vi "Main RT.vi"() -> ()   [LabVIEW 2021]
uses:
  <vilib>/FPGAPlugInAG/myRIO-1900/niLvFpga_Open_myRIO-1900.vi
  <vilib>/rvi/interface/common/dynamic/niFpgaDynamicAddResources.vi
  <vilib>/FPGAPlugInAG/Dynamic/niLvFpga_Run_Dynamic.vi
  <vilib>/Utility/error.llb/Error Cluster From Error Code.vi
  <vilib>/rvi/errors/niLvFpgaAdjustHostInterfaceError.vi
  <vilib>/FPGAPlugInAG/Dynamic/niLvFpga_Close_Dynamic.vi
  <vilib>/rvi/interface/nirviOpenFPGA/nirviOpenFPGA.xnode
  FPGA Bitfiles/tdmsproject_FPGATarget_MainFPGA_3ScZJD+QSjs.lvbitx
  <vilib>/rvi/interface/nirviMethod/nirviMethod.xnode
  <vilib>/rvi/interface/nirviReadWriteControl/nirviReadWriteControl.xnode
  <vilib>/rvi/interface/nirviCloseFPGA/nirviCloseFPGA.xnode
  NiFpgaLv.dll
  <vilib>/rvi/interface/Simulation/niFpgaSimulationCallBeginRW.vi
panel:
  in  "LED0":bool
  in  "stop":bool
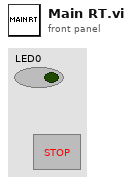
[diagram p1: front panel]
types:
  T1 = enum16{"open", "open or create", "create or replace", "create", "open (read-only)"}
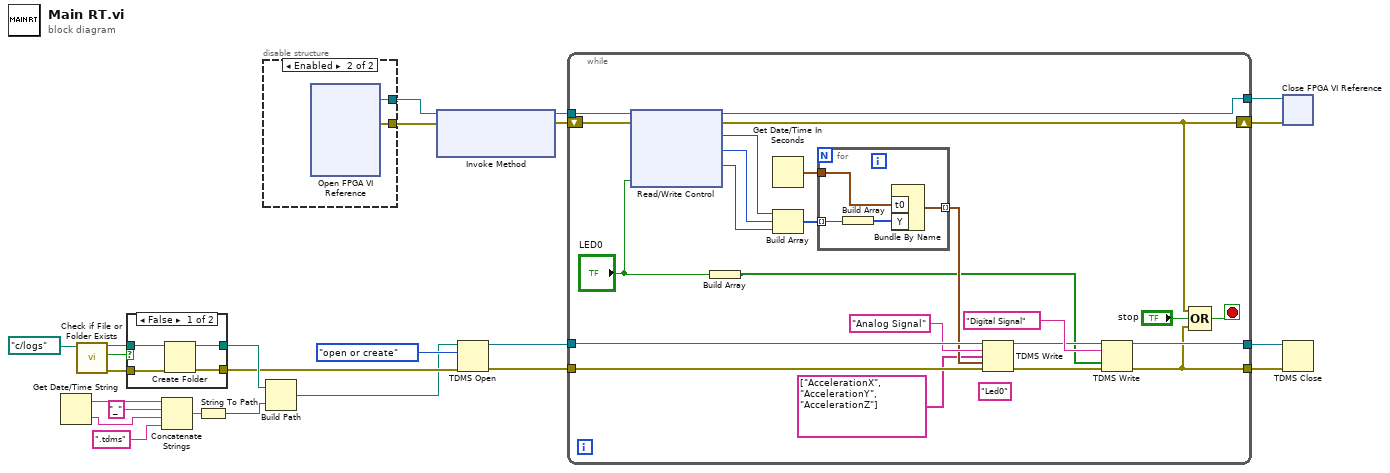
[diagram p0: block diagram]
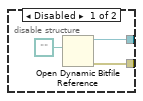
[diagram p3: hidden frame]
diagram:
  n1 = Get Date/Time String() -> (date string=w6:string, time string=w4:string)  [unwired: 3 in]
  n2 = call <vilib>:"Check if File or Folder Exists.vi"("path"=path "c:/logs" ("file path")) -> ("error out"=w10:errorcluster, "file or folder exists?"=w11:bool, "dup path"=w12:path)  [unwired: 8 in]
  n3 = case shown="False" w11 {
    tunnel: w12 -> [w28 w30]
    tunnel: [w27 w30] -> w9
    tunnel: [w26 w29] -> w8
    tunnel: w10 -> [w25 w29]
    frame False {
      n4 = Create Folder(path (use dialog)=w28, error in=w25) -> (created path=w27:path, error out=w26:errorcluster)  [unwired: 1 in, 1 out]
    }
    frame True {
    }
  }
  n5 = Concatenate Strings(w6, "_" ("string"), w4, ".tdms" ("string")) -> (w3:string)
  n6 = String To Path(string=w3) -> (path=w1:path)
  n7 = disable-structure shown="Enabled" {
    disable-tunnel: [w33 w34] -> w23
    disable-tunnel: [w32 w35] -> w22
    frame Disabled {
      n8 = Open Dynamic Bitfile Reference(1:path "" ("Bitfile path")) -> (5:w33:refnum<k20>, 8:w32:errorcluster)  [unwired: 4 in]
    }
    frame Enabled {
      n9 = xnode "Open FPGA VI Reference"() -> ("FPGA VI Reference Out"=w34:refnum<k20>, "error out"=w35:errorcluster)  [unwired: 2 in]
    }
  }
  n10 = Build Path(base path=w9, name or relative path=w1) -> (appended path=w7:path)
  n11 = xnode "Invoke Method"("FPGA VI Reference In"=w23, "error in"=w22) -> ("FPGA VI Reference Out"=w24:refnum<k20>, "error out"=w21:errorcluster)  [unwired: 1 in]
  n12 = TDMS Open(8:w8, 10:T1."open or create" ("operation (0:open)"), 11:w7) -> (0:w17:errorcluster, 3:w18:refnum<k34>)  [unwired: 4 in]
  n13 = while {
    tunnel: w24 -> [w58]
    shift-right: [w38] -> w20
    shift-left: w21 -> [w57]
    tunnel: [w56] -> w19
    tunnel: w18 -> [w55]
    tunnel: w17 -> [w54]
    tunnel: [w50] -> w16
    tunnel: [w36] -> w15
    stop <- w39 stop-if-true
    (unwired) "Led0" ("channel name(s) in (Untitled)")
    n14 = xnode "Read/Write Control"("FPGA VI Reference In"=w58, "error in"=w57, "LED0"="LED0") -> ("FPGA VI Reference Out"=w56:refnum<k20>, "error out"=w38:errorcluster, "AccelerationX"=w48:i16, "AccelerationY"=w47:i16, "AccelerationZ"=w43:i16)
    n15 = Build Array("LED0") -> (w41:bool[])
    n16 = Get Date/Time In Seconds() -> (seconds since 1Jan1904=w44:timestamp)
    n17 = Build Array(w48, w47, w43) -> (w46:i16[])
    n18 = for {
      tunnel: w46 -> [w60] mode=indexing
      tunnel: [w62] -> w45 mode=indexing
      tunnel: w44 -> [w61]
      n19 = Build Array(w60) -> (w59:i16[])
      n20 = Bundle By Name("t0"=w61, "Y"=w59) -> (w62:waveform(i16))  [unwired: 1 in]
    }
    n21 = TDMS Write(0:w55, 5:"Analog Signal" ("group name in (Untitled)"), 7:string[] ["AccelerationX", "AccelerationY", "AccelerationZ"] ("channel name(s) in (Untitled)"), 9:w45, 11:w54) -> (4:w49:refnum<k34>, 15:w51:errorcluster)  [unwired: 1 in, 2 out]
    n22 = TDMS Write(0:w49, 5:"Digital Signal" ("group name in (Untitled)"), 9:w41, 11:w51) -> (4:w50:refnum<k34>, 15:w36:errorcluster)  [unwired: 2 in, 2 out]
    n23 = Compound Arithmetic op=OR(w38, "stop", w36) -> (w39:bool)
  }
  n24 = xnode "Close FPGA VI Reference"("FPGA VI Reference In"=w19, "error in"=w20) -> ()  [unwired: 1 out]
  n25 = TDMS Close(8:w15, 11:w16) -> ()  [unwired: 2 out]
